vi "signal_simulator.vi"() -> ()   [LabVIEW 2023]
uses:
  <vilib>/express/express analysis/Spectral/Block/exnSpectralBlock spectral measurements RMS poly.vi
  <vilib>/express/express analysis/Spectral/Block/exnSpectralBlock spectral measurements RMS DDT.vi
  <vilib>/express/express analysis/Spectral/XNode/ExpressSpectralMeasurementsBlockNode.xnode
panel:
  in  "Start/Stop\nRecording":bool
  out "Recorded FFT":dynamicdata(graph)
  in  "Waves":T1(array[cluster]) {"Amplitude" scale=0.0..10.0; "Freq" scale=0.0..1000.0}
  in  "Apply Preset":bool
  in  "Preset":u16(ring) items=["Bells", "Brass"]
  in  "Clear Values":bool
  in  "Filter Cutoff Frequency":dbl(slide) scale=10.0..1000.0
  in  "Filter":T2(ring)
  in  "stop":bool
  in  "Sound On/Off":bool
  out "FFT  of Compound Signal":dynamicdata(graph) caption="FFT of Compound Signal"
  out "Raw Compond Signal":dynamicdata(graph)
  # "PRESETS"
  # "Compound Signal FFT"
  # "Raw Compound Signal"
  # "Recorded Signal FFT"
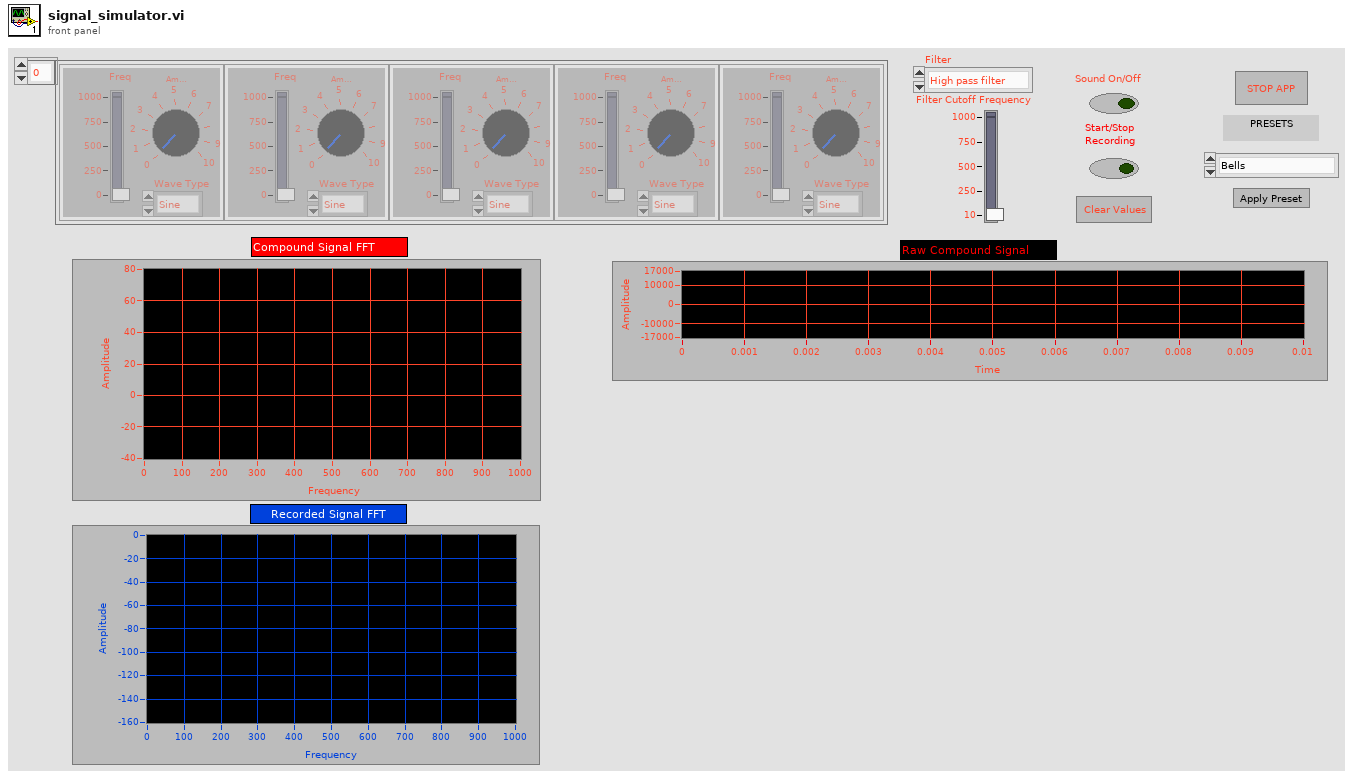
[diagram p1: front panel]
types:
  T1 = cluster{"Freq":dbl, "Amplitude":dbl, "Wave Type":enum16{"Sine", "Square", "Triangle", "Sawtooth"}}[]
  T2 = enum16{"High pass filter", "Low pass filter", "Filter off"}
  T3 = cluster{"averaging mode":u16, "weighting mode":u16, "number of averages":u32}
  T4 = cluster{"dB On (F)":bool, "unwrap phase (F)":bool, "convert to degree (F)":bool}
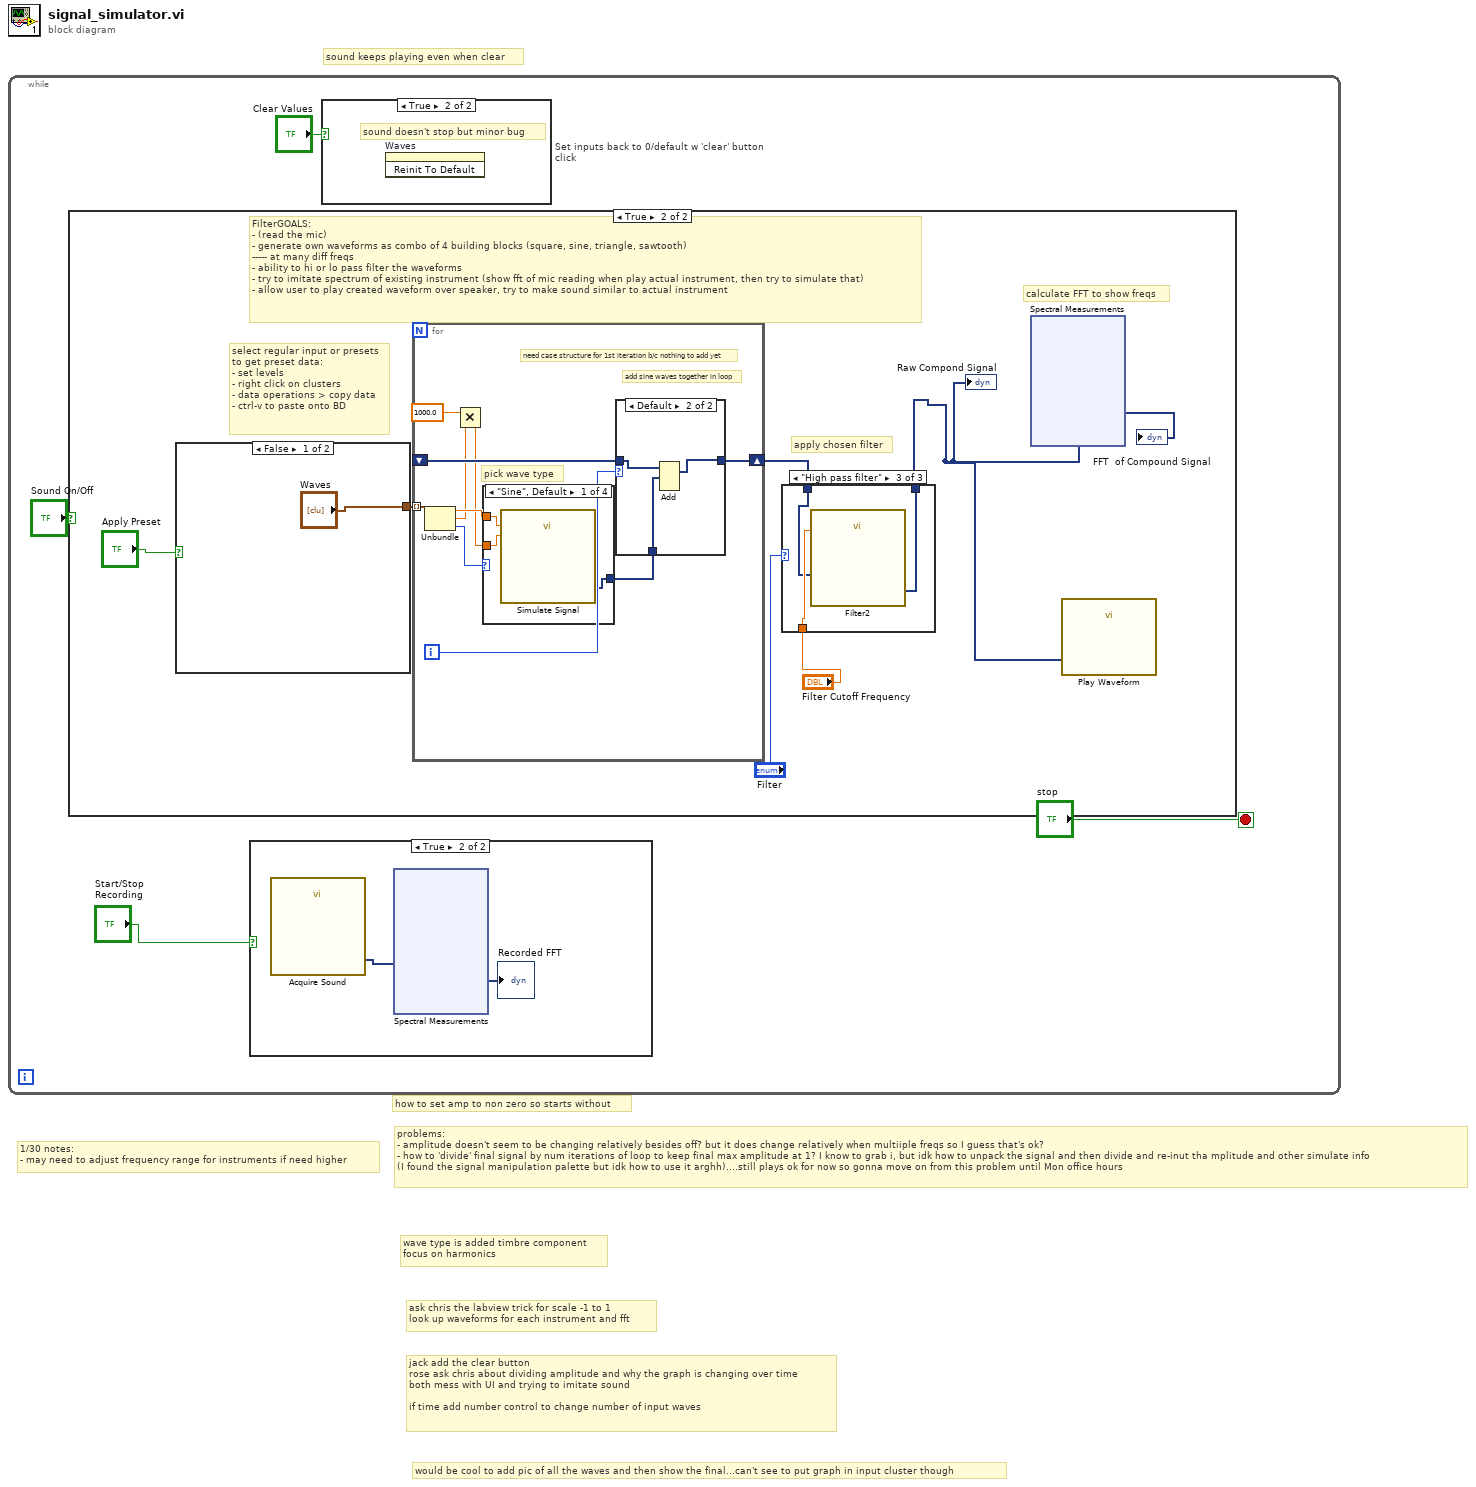
[diagram p0: block diagram]
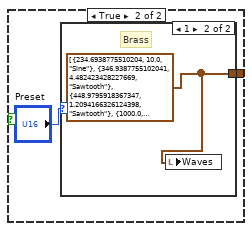
[diagram p5: hidden frame]
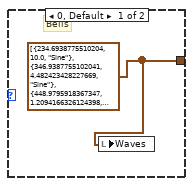
[diagram p6: hidden frame]
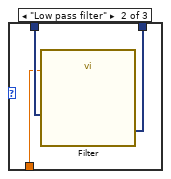
[diagram p8: hidden frame]
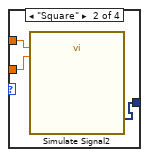
[diagram p9: hidden frame]
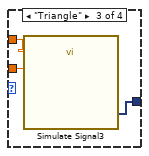
[diagram p10: hidden frame]
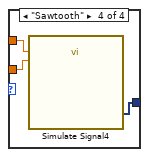
[diagram p11: hidden frame]
diagram:
  # "1/30 notes:\n- may need to adjust frequency range for instruments if need higher"
  # "would be cool to add pic of all the waves and then show the final...can't see to put graph in input cluster though"
  # "sound keeps playing even when clear"
  # "jack add the clear button\nrose ask chris about dividing amplitude and why the graph is changing over time\nboth mess with UI and trying to imitate sound\n\nif time add number control to change number of input waves"
  # "ask chris the labview trick for scale -1 to 1\nlook up waveforms for each instrument and fft"
  # "wave type is added timbre component\nfocus on harmonics"
  # "how to set amp to non zero so starts without"
  # "problems:\n- amplitude doesn't seem to be changing relatively besides off? but it does change relatively when multiiple freqs so I guess that's ok?\n- how to 'divide' final signal by num iterations of loop to keep final max amplitude at 1? I know to grab i, but idk how to unpack the signal and then divide and re-inut tha mplitude and other simulate info\n(I found the signal manipulation palette but idk how to use it arghh)....still plays ok for now so gonna move on from this problem until Mon office hours"
  n1 = while {
    stop <- "stop" stop-if-true
    n2 = case shown="True" "Sound On/Off" {
      frame False {
      }
      frame True {
        # "select regular input or presets\nto get preset data:\n- set levels\n- right click on clusters\n- data operations > copy data\n- ctrl-v to paste onto BD"
        # "calculate FFT to show freqs"
        # "apply chosen filter"
        # "FilterGOALS:\n- (read the mic)\n- generate own waveforms as combo of 4 building blocks (square, sine, triangle, sawtooth)\n----- at many diff freqs\n- ability to hi or lo pass filter the waveforms\n- try to imitate spectrum of existing instrument (show fft of mic reading when play actual instrument, then try to simulate that)\n- allow user to play created waveform over speaker, try to make sound similar to actual instrument"
        n3 = case shown="False" "Apply Preset" {
          tunnel: ["Waves" w26] -> w22
          frame False {
          }
          frame True {
            n4 = case shown="1" "Preset" {
              tunnel: [w27 w28] -> w26
              frame 0, Default {
                w27 = T1 [{"Freq"=234.6938775510204, "Amplitude"=10.0, "Wave Type"=enum."Sine"}, {"Freq"=346.9387755102041, "Amplitude"=4.482423428227669, "Wave Type"=enum."Sine"}, {"Freq"=448.9795918367347, "Amplitude"=1.2094166326124398, "Wave Type"=enum."Square"}, {"Freq"=1000.0, "Amplitude"=0.37360166242457055, "Wave Type"=enum."Square"}] ("Waves")
                # "Bells"
                n5 = local write "Waves"(w27) -> ()
              }
              frame 1 {
                w28 = T1 [{"Freq"=234.6938775510204, "Amplitude"=10.0, "Wave Type"=enum."Sine"}, {"Freq"=346.9387755102041, "Amplitude"=4.482423428227669, "Wave Type"=enum."Sawtooth"}, {"Freq"=448.9795918367347, "Amplitude"=1.2094166326124398, "Wave Type"=enum."Sawtooth"}, {"Freq"=1000.0, "Amplitude"=0.37360166242457055, "Wave Type"=enum."Square"}] ("Waves")
                # "Brass"
                n6 = local write "Waves"(w28) -> ()
              }
            }
          }
        }
        n7 = for {
          shift-right: [w55] -> w20
          shift-left: _ -> [w54]
          tunnel: w22 -> [w53] mode=indexing
          i -> [w51]
          # "pick wave type"
          # "need case structure for 1st iteration b/c nothing to add yet"
          # "add sine waves together in loop"
          n8 = Unbundle(w53) -> ("Freq"=w52:dbl, "Amplitude"=w49:dbl, "Wave Type"=w50:enum16{"Sine", "Square", "Triangle", "Sawtooth"})
          n9 = Multiply(x=1000.0, y=w49) -> (x*y=w47:dbl)
          n10 = case shown="\"Sine\", Default" w50 {
            tunnel: [w57 w60 w63 w66] -> w46
            tunnel: w52 -> [w58 w61 w64 w67]
            tunnel: w47 -> [w56 w59 w62 w65]
            frame "Sine", Default {
              n11 = call "Simulate Signal"("Frequency"=w58, "Amplitude"=w56) -> ("Sine"=w57:dynamicdata)  [unwired: 12 in, 1 out]
            }
            frame "Square" {
              n12 = call "Simulate Signal2"("Frequency"=w61, "Amplitude"=w59) -> ("Square"=w60:dynamicdata)  [unwired: 12 in, 1 out]
            }
            frame "Triangle" {
              n13 = call "Simulate Signal3"("Frequency"=w64, "Amplitude"=w62) -> ("Triangle"=w63:dynamicdata)  [unwired: 12 in, 1 out]
            }
            frame "Sawtooth" {
              n14 = call "Simulate Signal4"("Frequency"=w67, "Amplitude"=w65) -> ("Sawtooth"=w66:dynamicdata)  [unwired: 12 in, 1 out]
            }
          }
          n15 = case shown="Default" w51 {
            tunnel: w46 -> [w68 w71]
            tunnel: [w68 w70] -> w55
            tunnel: w54 -> [_ w69]
            frame 0 {
            }
            frame Default {
              n16 = Add(1:w71, 2:w69) -> (0:w70:dynamicdata)  [unwired: 1 in, 1 out]
            }
          }
        }
        n17 = case shown="\"High pass filter\"" "Filter" {
          tunnel: w20 -> [w29 w32 w34]
          tunnel: [w29 w31 w33] -> w18
          tunnel: "Filter Cutoff Frequency" -> [_ w30 w35]
          frame "Filter off" {
          }
          frame "Low pass filter" {
            n18 = call "Filter"("Lower Cut-Off"=w30, "Signal"=w32) -> ("Filtered Signal"=w31:dynamicdata)  [unwired: 8 in, 1 out]
          }
          frame "High pass filter" {
            n19 = call "Filter2"("Lower Cut-Off"=w35, "Signal"=w34) -> ("Filtered Signal"=w33:dynamicdata)  [unwired: 8 in, 1 out]
          }
        }
        "Raw Compond Signal" <- w18
        n20 = xnode "Spectral Measurements"("Signals"=w18) -> ("FFT - (RMS)"=→"FFT  of Compound Signal":dynamicdata)  [unwired: 1 in, 2 out]
        n21 = call "Play Waveform"("Data"=w18) -> ()  [unwired: 18 in, 1 out]
      }
    }
    n22 = case shown="True" "Start/Stop\nRecording" {
      frame False {
      }
      frame True {
        n23 = call "Acquire Sound"() -> ("Data"=w6:dynamicdata)  [unwired: 18 in, 1 out]
        n24 = xnode "Spectral Measurements"("Signals"=w6) -> ("FFT - (RMS)"=→"Recorded FFT":dynamicdata)  [unwired: 1 in, 2 out]
      }
    }
    n25 = case "Set inputs back to 0/default w 'clear' button click" shown="True" "Clear Values" {
      frame False {
      }
      frame True {
        # "sound doesn't stop but minor bug"
        n26 = invoke on="Waves" class="Arr (strict)" method="Reinit To Default"() -> ()  [unwired: 3 in, 3 out]
      }
    }
  }
